vi "PhotonPoseEstimator_Execute_LowestAmbiguity.vi"(7 "Configuration":T11={"Primary Strategy"=enum."LOWEST_AMBIGUITY", "Camera"="", "Initial Pose"={"Translation3d"={"X"=0.0, "Y"=0.0, "Z"=0.0}, "Rotation3d"={"Q_quaternion"={"R"=1.0, "V"=[0.0, 0.0, 0.0]}}}, "HighestAmbiguity"=0.0, "RobotToCamera"={"TRANSLATION3D"={"X"=0.0, "Y"=0.0, "Z"=0.0}, "ROTATION3D"={"Q_quaternion"={"R"=1.0, "V"=[0.0, 0.0, 0.0]}}, "XF"=FALSE}, "FallBack Strategy"=enum."LOWEST_AMBIGUITY", "BaseNTName"="/photonvision"} {"RobotToCamera"."TRANSLATION3D"."Z" format="%14.3f"; "RobotToCamera"."TRANSLATION3D"."Y" format="%14.3f"; "RobotToCamera"."TRANSLATION3D"."X" format="%14.3f"; "Initial Pose"."Translation3d"."Z" format="%14.3f"; "Initial Pose"."Translation3d"."Y" format="%14.3f"; "Initial Pose"."Translation3d"."X" format="%14.3f"}, 8 "AprilTagFieldLayout":T1={"AprilTagMap"={}, "FieldLength"=0.0, "FieldWidth"=0.0, "OriginPosition "=enum."kBlueAllianceWallRightSide,", "OriginPose3d"={"Translation3d"={"X"=0.0, "Y"=0.0, "Z"=0.0}, "Rotation3d"={"Q_quaternion"={"R"=1.0, "V"=[0.0, 0.0, 0.0]}}}} {"OriginPose3d"."Translation3d"."Z" format="%14.3f"; "OriginPose3d"."Translation3d"."Y" format="%14.3f"; "OriginPose3d"."Translation3d"."X" format="%14.3f"}, 10 "PIpeline Has \nNew Results":bool, 11 "PipelineResult":T14={"Targets"=[], "PhotonMultiTargetPNPResult"={"PhotonPNPResult"={"IsPresent"=FALSE, "bestReprojErr"=0.0, "altReprojErr"=0.0, "ambiguity"=0.0, "Best"={"TRANSLATION3D"={"X"=0.0, "Y"=0.0, "Z"=0.0}, "ROTATION3D"={"Q_quaternion"={"R"=1.0, "V"=[0.0, 0.0, 0.0]}}, "XF"=FALSE}, "Alt"={"TRANSLATION3D"={"X"=0.0, "Y"=0.0, "Z"=0.0}, "ROTATION3D"={"Q_quaternion"={"R"=1.0, "V"=[0.0, 0.0, 0.0]}}, "XF"=FALSE}}, "FiducialIDsUsed"=[]}, "PhotonPipelineMetadata"={"CaptureTimestampMicros"=0, "PublishTimestampMicros"=0, "SequenceID"=0, "TimeSinceLastPong"=0}} {"PhotonMultiTargetPNPResult"."PhotonPNPResult"."Alt"."TRANSLATION3D"."Z" format="%14.3f"; "PhotonMultiTargetPNPResult"."PhotonPNPResult"."Alt"."TRANSLATION3D"."Y" format="%14.3f"; "PhotonMultiTargetPNPResult"."PhotonPNPResult"."Alt"."TRANSLATION3D"."X" format="%14.3f"; "PhotonMultiTargetPNPResult"."PhotonPNPResult"."Best"."TRANSLATION3D"."Z" format="%14.3f"; "PhotonMultiTargetPNPResult"."PhotonPNPResult"."Best"."TRANSLATION3D"."Y" format="%14.3f"; "PhotonMultiTargetPNPResult"."PhotonPNPResult"."Best"."TRANSLATION3D"."X" format="%14.3f"; "Targets"."AltCameraToTarget"."TRANSLATION3D"."Z" format="%14.3f"; "Targets"."AltCameraToTarget"."TRANSLATION3D"."Y" format="%14.3f"; "Targets"."AltCameraToTarget"."TRANSLATION3D"."X" format="%14.3f"; "Targets"."BestCameraToTarget"."TRANSLATION3D"."Z" format="%14.3f"; "Targets"."BestCameraToTarget"."TRANSLATION3D"."Y" format="%14.3f"; "Targets"."BestCameraToTarget"."TRANSLATION3D"."X" format="%14.3f"}) -> (0 "TimeStamp_Seconds":dbl, 1 "New Pose Found":bool, 2 "EstimatedPose2d":T8={"TRANSLATION"={"X"=0.0, "Y"=0.0}, "ROTATION"={"VALUE"=0.0, "COS"=1.0, "SIN"=0.0}} {"ROTATION"."SIN" format="%13.4f"; "ROTATION"."COS" format="%13.4f"; "ROTATION"."VALUE" format="%13.4f"; "TRANSLATION"."Y" format="%14.3f"; "TRANSLATION"."X" format="%14.3f"}, 3 "EstimatedPose3d":T3={"Translation3d"={"X"=0.0, "Y"=0.0, "Z"=0.0}, "Rotation3d"={"Q_quaternion"={"R"=1.0, "V"=[0.0, 0.0, 0.0]}}} {"Translation3d"."Z" format="%14.3f"; "Translation3d"."Y" format="%14.3f"; "Translation3d"."X" format="%14.3f"}, 5 "PhotonEstimatedRobotPose":T20={"EstimatedPose"={"Translation3d"={"X"=0.0, "Y"=0.0, "Z"=0.0}, "Rotation3d"={"Q_quaternion"={"R"=1.0, "V"=[0.0, 0.0, 0.0]}}}, "TimeStamp_Seconds"=0.0, "targetsUsed"=[], "Strategy"=enum."LOWEST_AMBIGUITY"} {"targetsUsed"."AltCameraToTarget"."TRANSLATION3D"."Z" format="%14.3f"; "targetsUsed"."AltCameraToTarget"."TRANSLATION3D"."Y" format="%14.3f"; "targetsUsed"."AltCameraToTarget"."TRANSLATION3D"."X" format="%14.3f"; "targetsUsed"."BestCameraToTarget"."TRANSLATION3D"."Z" format="%14.3f"; "targetsUsed"."BestCameraToTarget"."TRANSLATION3D"."Y" format="%14.3f"; "targetsUsed"."BestCameraToTarget"."TRANSLATION3D"."X" format="%14.3f"; "EstimatedPose"."Translation3d"."Z" format="%14.3f"; "EstimatedPose"."Translation3d"."Y" format="%14.3f"; "EstimatedPose"."Translation3d"."X" format="%14.3f"}, 6 "out PhotonPoseEstimator":T21={"LastPose"={"Translation3d"={"X"=0.0, "Y"=0.0, "Z"=0.0}, "Rotation3d"={"Q_quaternion"={"R"=1.0, "V"=[0.0, 0.0, 0.0]}}}, "ReferencePose"={"Translation3d"={"X"=0.0, "Y"=0.0, "Z"=0.0}, "Rotation3d"={"Q_quaternion"={"R"=1.0, "V"=[0.0, 0.0, 0.0]}}}, "FieldTags"={"AprilTagMap"={}, "FieldLength"=0.0, "FieldWidth"=0.0, "OriginPosition "=enum."kBlueAllianceWallRightSide,", "OriginPose3d"={"Translation3d"={"X"=0.0, "Y"=0.0, "Z"=0.0}, "Rotation3d"={"Q_quaternion"={"R"=1.0, "V"=[0.0, 0.0, 0.0]}}}}, "PrimaryStratety"=enum."LOWEST_AMBIGUITY", "Camera"="", "RobotToCamera"={"TRANSLATION3D"={"X"=0.0, "Y"=0.0, "Z"=0.0}, "ROTATION3D"={"Q_quaternion"={"R"=1.0, "V"=[0.0, 0.0, 0.0]}}, "XF"=FALSE}, "ReportedErrors"=[], "HighestAmbiguity"=10.0, "MultiTagFallbackStrategy"=enum."LOWEST_AMBIGUITY", "PoseCacheTimeoutSec"=-1.0, "PhotonTargetModel"={"Vertices"=[], "IsPlaner"=FALSE, "IsSpherical"=FALSE}, "BaseNTName"="/photonvision"} {"PhotonTargetModel"."Vertices"."Z" format="%14.3f"; "PhotonTargetModel"."Vertices"."Y" format="%14.3f"; "PhotonTargetModel"."Vertices"."X" format="%14.3f"; "RobotToCamera"."TRANSLATION3D"."Z" format="%14.3f"; "RobotToCamera"."TRANSLATION3D"."Y" format="%14.3f"; "RobotToCamera"."TRANSLATION3D"."X" format="%14.3f"; "FieldTags"."OriginPose3d"."Translation3d"."Z" format="%14.3f"; "FieldTags"."OriginPose3d"."Translation3d"."Y" format="%14.3f"; "FieldTags"."OriginPose3d"."Translation3d"."X" format="%14.3f"; "ReferencePose"."Translation3d"."Z" format="%14.3f"; "ReferencePose"."Translation3d"."Y" format="%14.3f"; "ReferencePose"."Translation3d"."X" format="%14.3f"; "LastPose"."Translation3d"."Z" format="%14.3f"; "LastPose"."Translation3d"."Y" format="%14.3f"; "LastPose"."Translation3d"."X" format="%14.3f"})   [LabVIEW 2019, in "PhotonVisionLib.lvlib"]
doc: "Provided data from polling a camera, update the estimated position of the robot. Returns empty if there are no cameras set or no targets were found from the cameras. \n\nInputs:\n -- PhotonPoseEstimator -- data cluster -- Data guiding how the position determination is done.\n -- PipelineResults -- data cluster -- Data provided from PhotonCamera_GetLatestResults.\n -- HasResults -- boolean - TRUE if targets have been identified in the Pipeline results. This can be provided by PhotonCamera_GetLatestResults.\n -- AprilTagFieldLayout -- data cluster -- Field layout defining the location of April Tags\n\nOutputs:\n - EstimatedPose3d - Pose3d - Estimated 3d position. Only value if NewPoseFound = TRUE\n - EstimatedPose2d - Pose2d - Estimated 2d position. Only value if NewPoseFound = TRUE\n - NewPoseFound -- boolean -- A new position has been determined.\n - TimeStampe - double - Target timestamp (seconds)\n - StrategyUsed -- enum -- The strategy used to determine the pose.\n - PhotonEstimatedRobotPose -- data cluster -- Complete estimated robot position and timestamp data cluster\n -- PhotonPoseEstimator -- data cluster -- Updated data cluster."
uses:
  PhotonVisionLib.lvlib
  <vilib>/Rock Robotics/WPI/ThirdParty/JAS_Junk/TrajLib/Trajectory_Library.lvlib
  <vilib>/Rock Robotics/WPI/ThirdParty/JAS_Junk/TrajLib/TypeDef/TRANSLATION3D.ctl
  <vilib>/Rock Robotics/WPI/ThirdParty/JAS_Junk/TrajLib/TypeDef/QUATERNION.ctl
  <vilib>/Rock Robotics/WPI/ThirdParty/JAS_Junk/TrajLib/TypeDef/ROTATION3D.ctl
  <vilib>/Rock Robotics/WPI/ThirdParty/JAS_Junk/TrajLib/TypeDef/TRANSFORM3D.ctl
  <vilib>/Rock Robotics/WPI/ThirdParty/JAS_Junk/TrajLib/TypeDef/POSE3D.ctl
  <vilib>/Rock Robotics/WPI/ThirdParty/JAS_Junk/TrajLib/TypeDef/AprilTag.ctl
  <vilib>/Rock Robotics/WPI/ThirdParty/JAS_Junk/TrajLib/Enum/AprilTagFieldLayoutOrignPosition_ENUM.ctl
  <vilib>/Rock Robotics/WPI/ThirdParty/JAS_Junk/TrajLib/TypeDef/AprilTagFieldLayout.ctl
  Enum/PhotonPoseStrategy_ENUM.ctl
  TypeDef/PhotonPoseEstimatorType.ctl
  TypeDef/PhotonEstimatedRobotPoseType.ctl
  TypeDef/TargetCornerType.ctl
  TypeDef/PhotonTrackedTargetType.ctl
  TypeDef/PhotonPipelineResultType.ctl
  TypeDef/PhotonPoseEstimator_Configuration.ctl
  TypeDef/PhotonPNPResultType.ctl
  TypeDef/PhotonMultiTargetPNPResultType.ctl
  TypeDef/PhotonTargetModel.ctl
  <vilib>/Rock Robotics/WPI/ThirdParty/JAS_Junk/TrajLib/TypeDef/TRANSLATION2D.ctl
  <vilib>/Rock Robotics/WPI/ThirdParty/JAS_Junk/TrajLib/TypeDef/ROTATION2D.ctl
  <vilib>/Rock Robotics/WPI/ThirdParty/JAS_Junk/TrajLib/TypeDef/POSE2D.ctl
  TypeDef/PhotonPipelineMetadataType.ctl
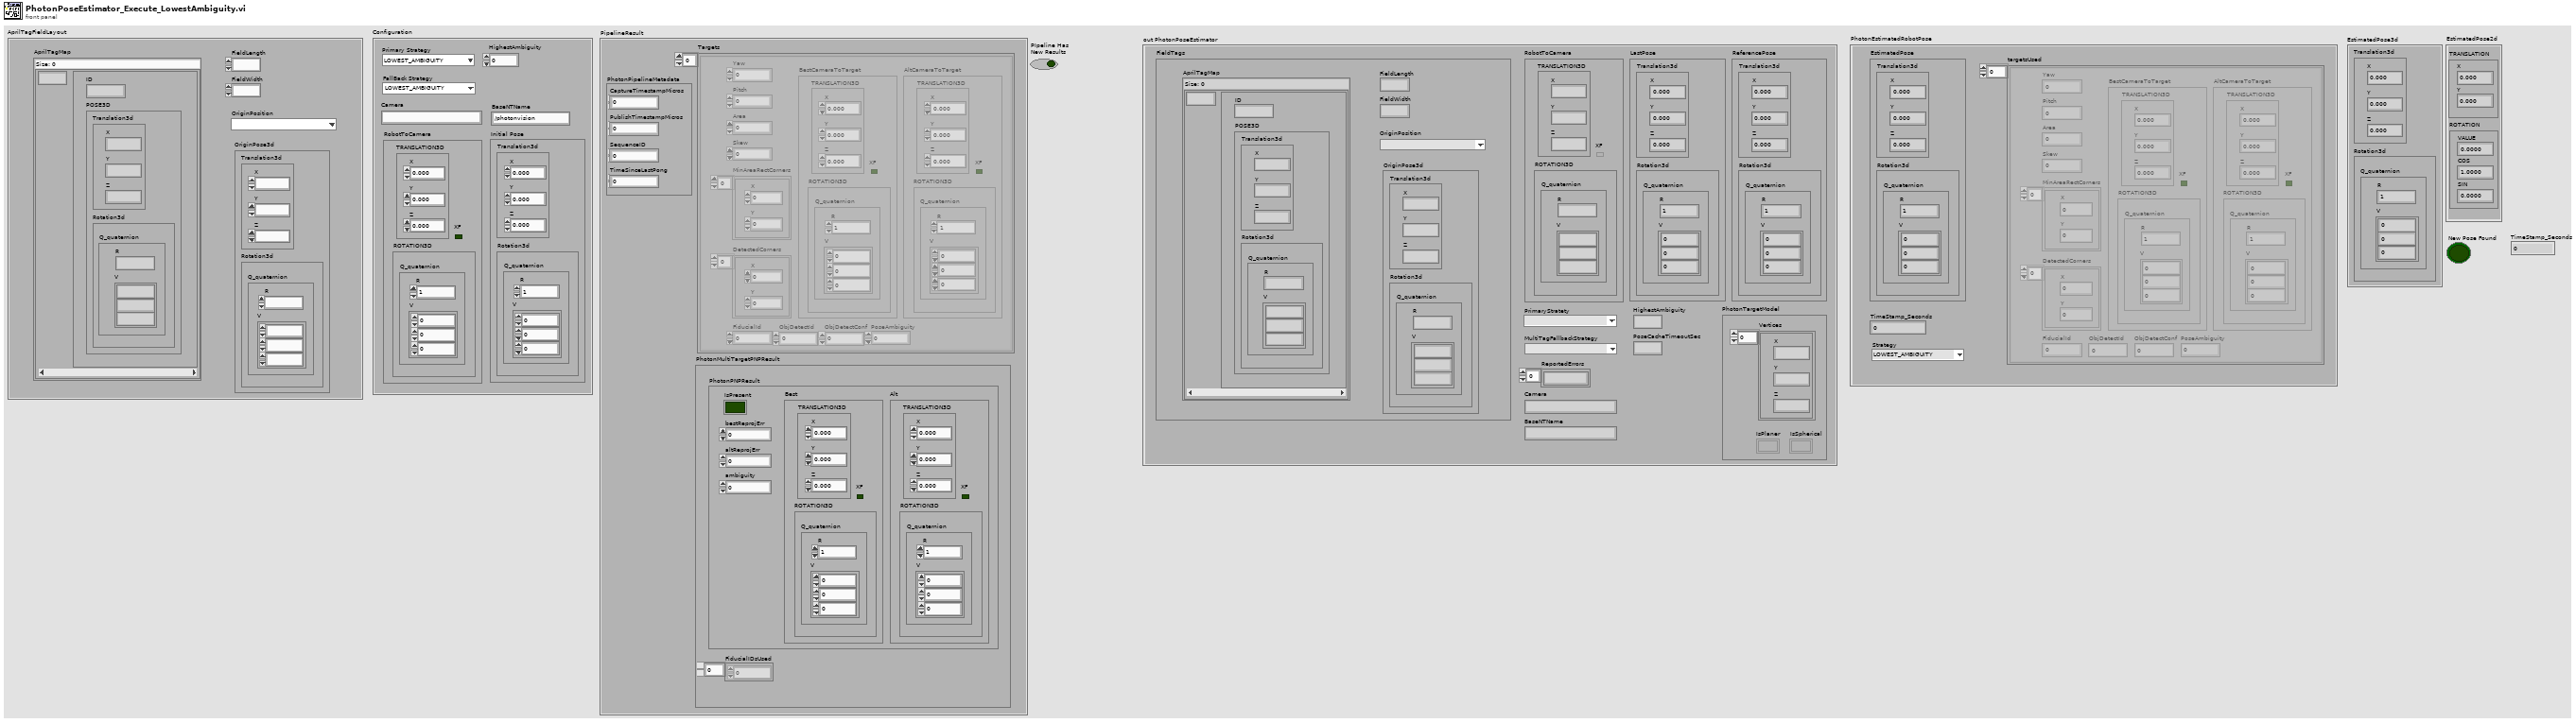
[diagram p1: front panel]
types:
  T1 = typedef "Trajectory_Library.lvlib/AprilTagFieldLayout.ctl" = cluster{"AprilTagMap":map{i32, T2}, "FieldLength":dbl, "FieldWidth":dbl, "OriginPosition ":T7, "OriginPose3d":T3}
  T2 = typedef "Trajectory_Library.lvlib/AprilTag.ctl" = cluster{"ID":i32, "POSE3D":T3}
  T3 = typedef "Trajectory_Library.lvlib/POSE3D.ctl" = cluster{"Translation3d":T4, "Rotation3d":T5}
  T4 = typedef "Trajectory_Library.lvlib/TRANSLATION3D.ctl" = cluster{"X":dbl, "Y":dbl, "Z":dbl}
  T5 = typedef "Trajectory_Library.lvlib/ROTATION3D.ctl" = cluster{"Q_quaternion":T6}
  T6 = typedef "Trajectory_Library.lvlib/QUATERNION.ctl" = cluster{"R":dbl, "V":dbl[]}
  T7 = typedef "Trajectory_Library.lvlib/AprilTagFieldLayoutOrignPosition_ENUM.ctl" = enum16{"kBlueAllianceWallRightSide,", "kRedAllianceWallRightSide,"}
  T8 = typedef "Trajectory_Library.lvlib/POSE2D.ctl" = cluster{"TRANSLATION":T9, "ROTATION":T10}
  T9 = typedef "Trajectory_Library.lvlib/TRANSLATION2D.ctl" = cluster{"X":dbl, "Y":dbl}
  T10 = typedef "Trajectory_Library.lvlib/ROTATION2D.ctl" = cluster{"VALUE":dbl, "COS":dbl, "SIN":dbl}
  T11 = typedef "PhotonVisionLib.lvlib/PhotonPoseEstimator_Configuration.ctl" = cluster{"Primary Strategy":T12, "Camera":string, "Initial Pose":T3, "HighestAmbiguity":dbl, "RobotToCamera":T13, "FallBack Strategy":T12, "BaseNTName":string}
  T12 = typedef "PhotonVisionLib.lvlib/PhotonPoseStrategy_ENUM.ctl" = enum16{"LOWEST_AMBIGUITY", "CLOSEST_TO_CAMERA_HEIGHT", "CLOSEST_TO_REFERENCE_POSE", "CLOSEST_TO_LAST_POSE", "AVERAGE_BEST_TARGETS", "MULTI_TAG_PNP_ON_COPROCESSOR", "MULTI_TAG_PNP_ON_RIO", "PNP_DISTANCE_TRIG_SOLVE", "CONSTRAINED_SOLVEPNP"}
  T13 = typedef "Trajectory_Library.lvlib/TRANSFORM3D.ctl" = cluster{"TRANSLATION3D":T4, "ROTATION3D":T5, "XF":bool}
  T14 = typedef "PhotonVisionLib.lvlib/PhotonPipelineResultType.ctl" = cluster{"Targets":T15[], "PhotonMultiTargetPNPResult":T17, "PhotonPipelineMetadata":T19}
  T15 = typedef "PhotonVisionLib.lvlib/PhotonTrackedTargetType.ctl" = cluster{"Yaw":dbl, "Pitch":dbl, "Area":dbl, "Skew":dbl, "MinAreaRectCorners":T16[], "BestCameraToTarget":T13, "FiducialId":i32, "AltCameraToTarget":T13, "PoseAmbiguity":dbl, "DetectedCorners":T16[], "ObjDetectId":i32, "ObjDetectConf":sgl}
  T16 = typedef "PhotonVisionLib.lvlib/TargetCornerType.ctl" = cluster{"X":dbl, "Y":dbl}
  T17 = typedef "PhotonVisionLib.lvlib/PhotonMultiTargetPNPResultType.ctl" = cluster{"PhotonPNPResult":T18, "FiducialIDsUsed":i16[]}
  T18 = typedef "PhotonVisionLib.lvlib/PhotonPNPResultType.ctl" = cluster{"IsPresent":bool, "bestReprojErr":dbl, "altReprojErr":dbl, "ambiguity":dbl, "Best":T13, "Alt":T13}
  T19 = typedef "PhotonVisionLib.lvlib/PhotonPipelineMetadataType.ctl" = cluster{"CaptureTimestampMicros":i64, "PublishTimestampMicros":i64, "SequenceID":i64, "TimeSinceLastPong":i64}
  T20 = typedef "PhotonVisionLib.lvlib/PhotonEstimatedRobotPoseType.ctl" = cluster{"EstimatedPose":T3, "TimeStamp_Seconds":dbl, "targetsUsed":T15[], "Strategy":T12}
  T21 = typedef "PhotonVisionLib.lvlib/PhotonPoseEstimatorType.ctl" = cluster{"LastPose":T3, "ReferencePose":T3, "FieldTags":T1, "PrimaryStratety":T12, "Camera":string, "RobotToCamera":T13, "ReportedErrors":dbl[], "HighestAmbiguity":dbl, "MultiTagFallbackStrategy":T12, "PoseCacheTimeoutSec":dbl, "PhotonTargetModel":T22, "BaseNTName":string}
  T22 = typedef "PhotonVisionLib.lvlib/PhotonTargetModel.ctl" = cluster{"Vertices":T4[], "IsPlaner":bool, "IsSpherical":bool}
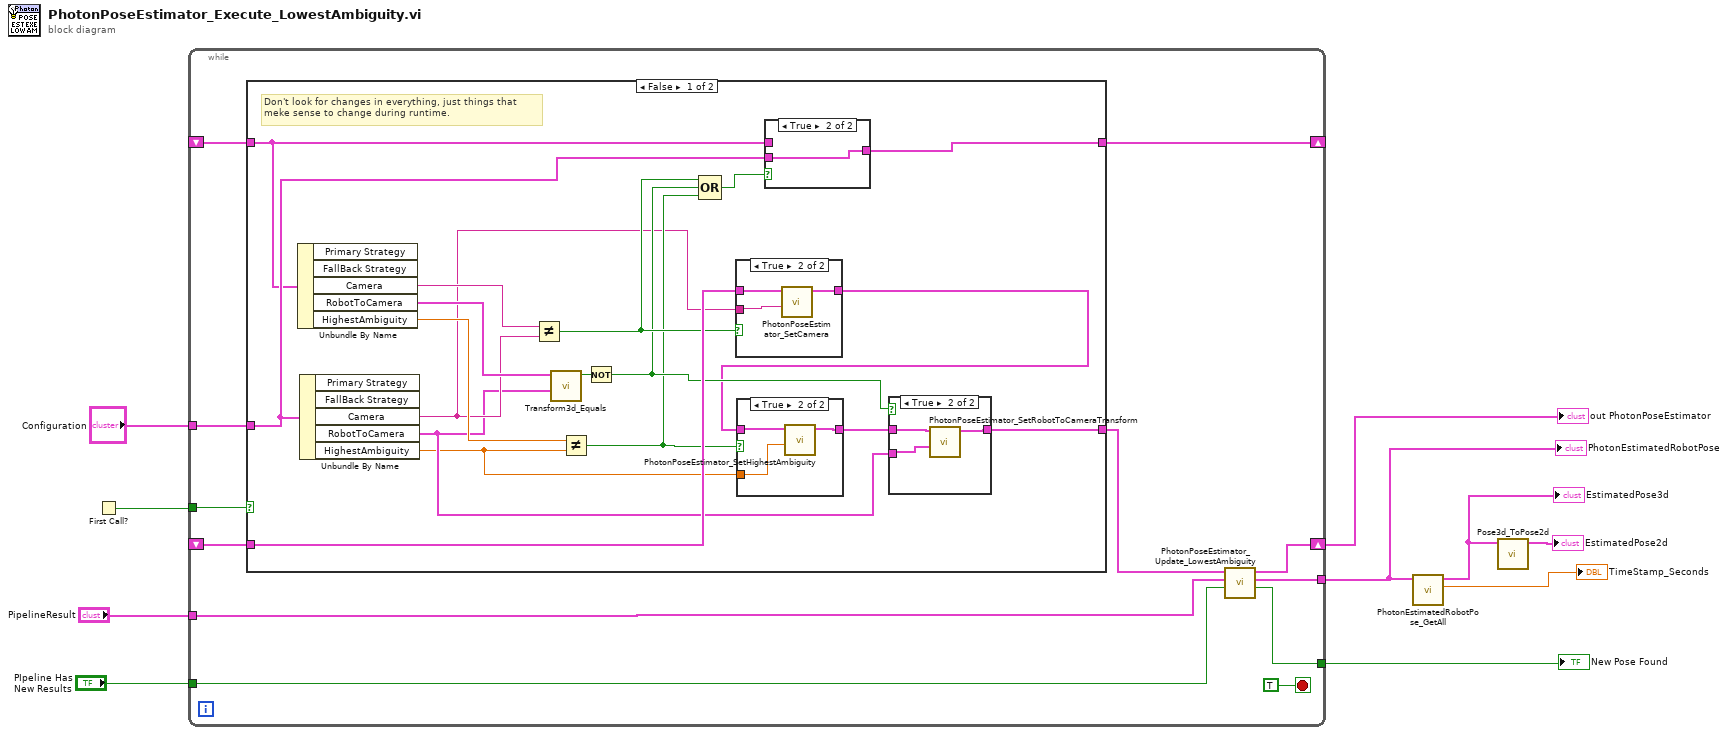
[diagram p0: block diagram]
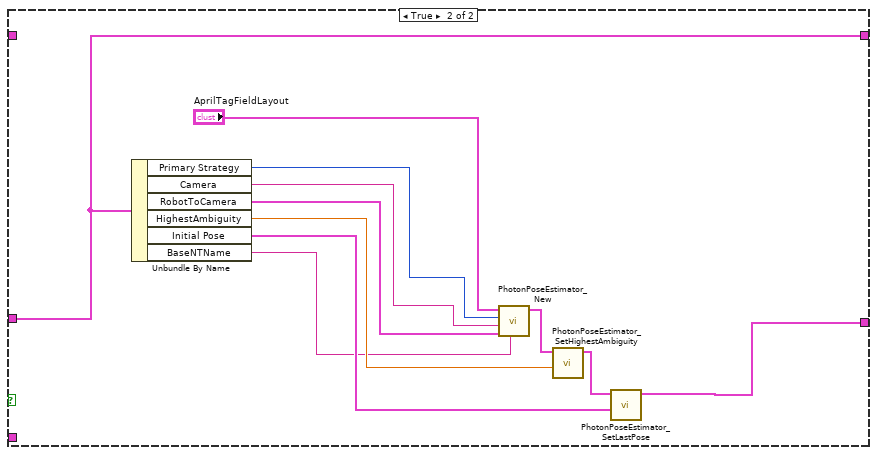
[diagram p6: hidden frame]
diagram:
  n1 = First Call?() -> (First Call?: T/F=w10:bool)
  n2 = while {
    tunnel: w10 -> [w12]
    tunnel: "PipelineResult" -> [w20]
    shift-right: [w18] -> w7
    shift-left: _ -> [w21]
    tunnel: "PIpeline Has \nNew Results" -> [w19]
    tunnel: [w17] -> w4
    tunnel: [w16] -> w6
    tunnel: "Configuration" -> [w14]
    shift-right: [w15] -> _
    shift-left: _ -> [w13]
    stop <- TRUE stop-if-true
    n3 = case shown="False" w12 {
      tunnel: [w24 w55] -> w11
      tunnel: w21 -> [w34 _]
      tunnel: w14 -> [w37 w58]
      tunnel: [w35 w58] -> w15
      tunnel: w13 -> [w36 _]
      frame False {
        # "Don't look for changes in everything, just things that\nmeke sense to change during runtime."
        n4 = Unbundle By Name(w36) -> ("Camera"=w32:string, "RobotToCamera"=w29:T13, "HighestAmbiguity"=w40:dbl)  [unwired: 2 out]
        n5 = Unbundle By Name(w37) -> ("Camera"=w27:string, "RobotToCamera"=w26:T13, "HighestAmbiguity"=w25:dbl)  [unwired: 2 out]
        n6 = Not Equal?(x=w32, y=w27) -> (x != y?=w33:bool)
        n7 = call <vilib>:"Transform3d_Equals.vi"("otherTransform3d"=w26, "inTransform3d"=w29) -> ("Equals"=w39:bool)  [unwired: 9 in]
        n8 = Not Equal?(x=w40, y=w25) -> (x != y?=w28:bool)
        n9 = Not(x=w39) -> (.not. x?=w30:bool)
        n10 = Compound Arithmetic op=OR(w33, w30, w28) -> (w38:bool)
        n11 = case shown="True" w33 {
          tunnel: w34 -> [w51 w54]
          tunnel: [w51 w53] -> w23
          tunnel: w27 -> [_ w52]
          frame False {
          }
          frame True {
            n12 = call "PhotonPoseEstimator_SetCamera.vi"("Camera"=w52, "PhotonPoseEstimator"=w54) -> ("out PhotonPoseEstimator"=w53:T21)  [unwired: 9 in]
          }
        }
        n13 = case shown="True" w28 {
          tunnel: w23 -> [w45 w48]
          tunnel: [w45 w47] -> w31
          tunnel: w25 -> [_ w46]
          frame False {
          }
          frame True {
            n14 = call "PhotonPoseEstimator_SetHighestAmbiguity.vi"("HighestAmbiguity"=w46, "PhotonPoseEstimator"=w48) -> ("out PhotonPoseEstimator"=w47:T21)  [unwired: 9 in]
          }
        }
        n15 = case shown="True" w38 {
          tunnel: w37 -> [_ w50]
          tunnel: w36 -> [w49 _]
          tunnel: [w49 w50] -> w35
          frame False {
          }
          frame True {
          }
        }
        n16 = case shown="True" w30 {
          tunnel: w31 -> [w41 w44]
          tunnel: [w41 w43] -> w24
          tunnel: w26 -> [_ w42]
          frame False {
          }
          frame True {
            n17 = call "PhotonPoseEstimator_SetRobotToCameraTransform.vi"("RobotToCameraTransform3d"=w42, "PhotonPoseEstimator"=w44) -> ("out PhotonPoseEstimator"=w43:T21)  [unwired: 9 in]
          }
        }
      }
      frame True {
        n18 = Unbundle By Name(w58) -> ("Primary Strategy"=w63:T12, "Camera"=w62:string, "RobotToCamera"=w61:T13, "HighestAmbiguity"=w60:dbl, "Initial Pose"=w59:T3, "BaseNTName"=w57:string)
        n19 = call "PhotonPoseEstimator_New.vi"("BaseNTName"=w57, "RobotToCamera"=w61, "Camera"=w62, "Strategy"=w63, "AprilTagFieldLayout"="AprilTagFieldLayout") -> ("PhotonPoseEstimator"=w65:T21)  [unwired: 6 in]
        n20 = call "PhotonPoseEstimator_SetHighestAmbiguity.vi"("HighestAmbiguity"=w60, "PhotonPoseEstimator"=w65) -> ("out PhotonPoseEstimator"=w64:T21)  [unwired: 9 in]
        n21 = call "PhotonPoseEstimator_SetLastPose.vi"("LastPose"=w59, "PhotonPoseEstimator"=w64) -> ("out PhotonPoseEstimator"=w55:T21)  [unwired: 9 in]
      }
    }
    n22 = call "PhotonPoseEstimator_Update_LowestAmbiguity.vi"("Has Results"=w19, "PipelineResult"=w20, "PhotonPoseEstimator"=w11) -> ("Pos Found"=w16:bool, "PhotonEstimatedRobotPose"=w17:T20, "out PhotonPoseEstimator"=w18:T21)  [unwired: 6 in]
  }
  "out PhotonPoseEstimator" <- w7
  "PhotonEstimatedRobotPose" <- w4
  "New Pose Found" <- w6
  n23 = call "PhotonEstimatedRobotPose_GetAll.vi"("PhotonEstimatedRobotPose"=w4) -> ("TimeStamp_Seconds"=→"TimeStamp_Seconds":dbl, "EstimatedPose"=w3:T3)  [unwired: 7 in, 2 out]
  "EstimatedPose3d" <- w3
  n24 = call <vilib>:"Pose3d_ToPose2d.vi"("in Pose3d"=w3) -> ("out Pose2d"=→"EstimatedPose2d":T8)  [unwired: 10 in]
